vi "Save PDF files.vi"(6 "Duplicate Plot":bool, 7 "Open in Acrobat":bool, 9 "Desired Filename":string, 10 "Data Directories":string[](array[string]), 11 "PDF file in":path) -> (1 "Saved Files":path[](array[path]), 3 "Results Folders":path[](array[path]))   [LabVIEW 2021]
uses:
  Globals/Constants_global.vi
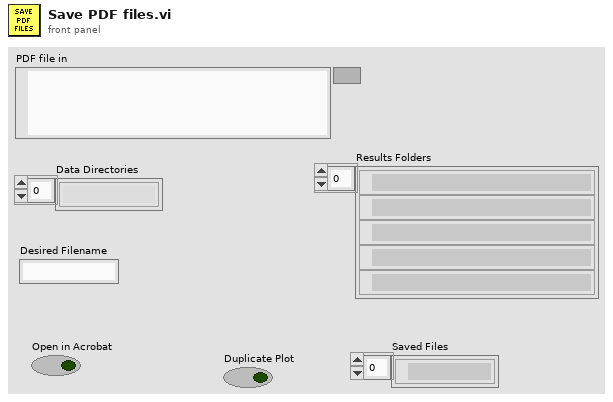
[diagram p1: front panel]
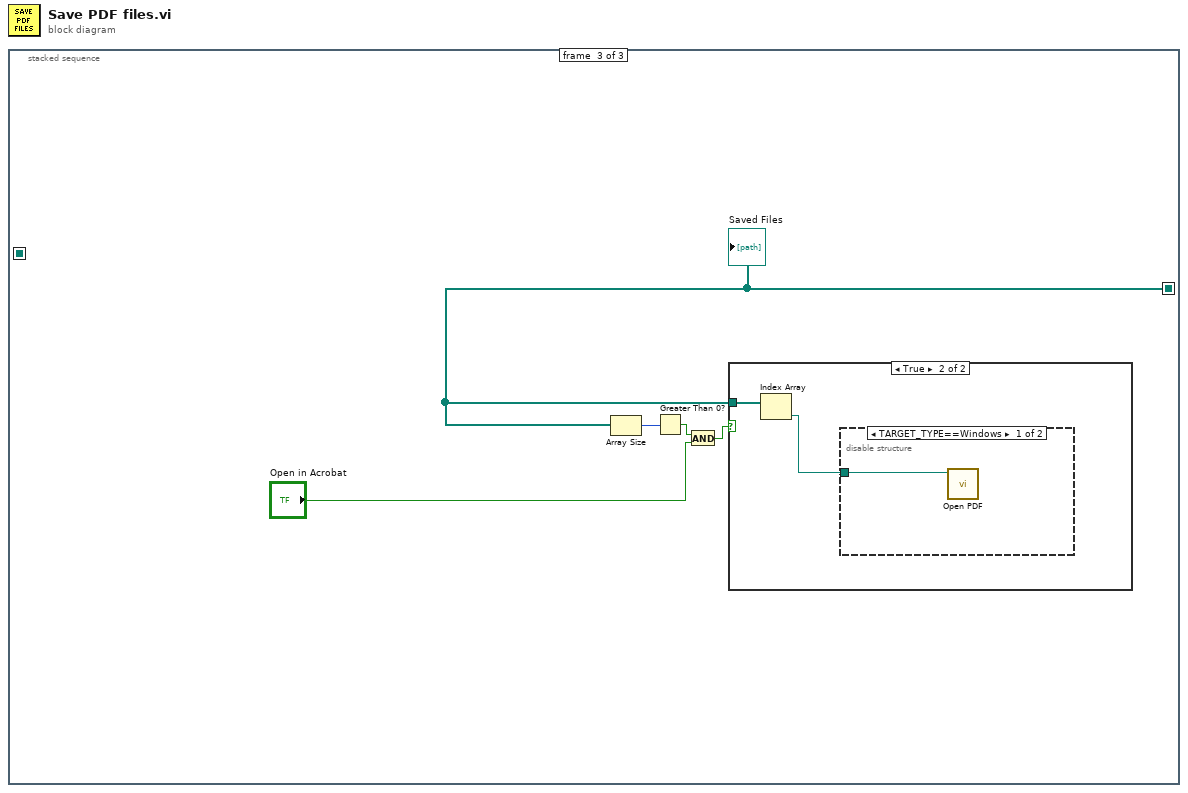
[diagram p0: block diagram]
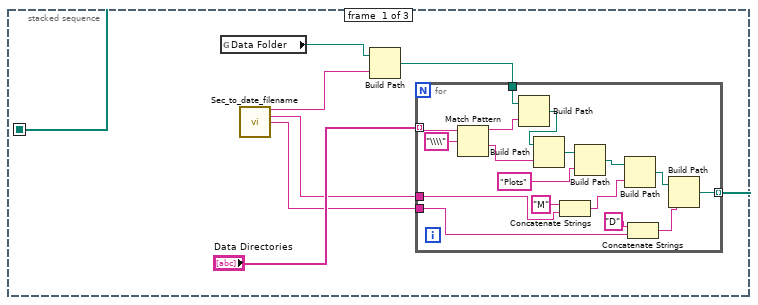
[diagram p2: hidden frame]
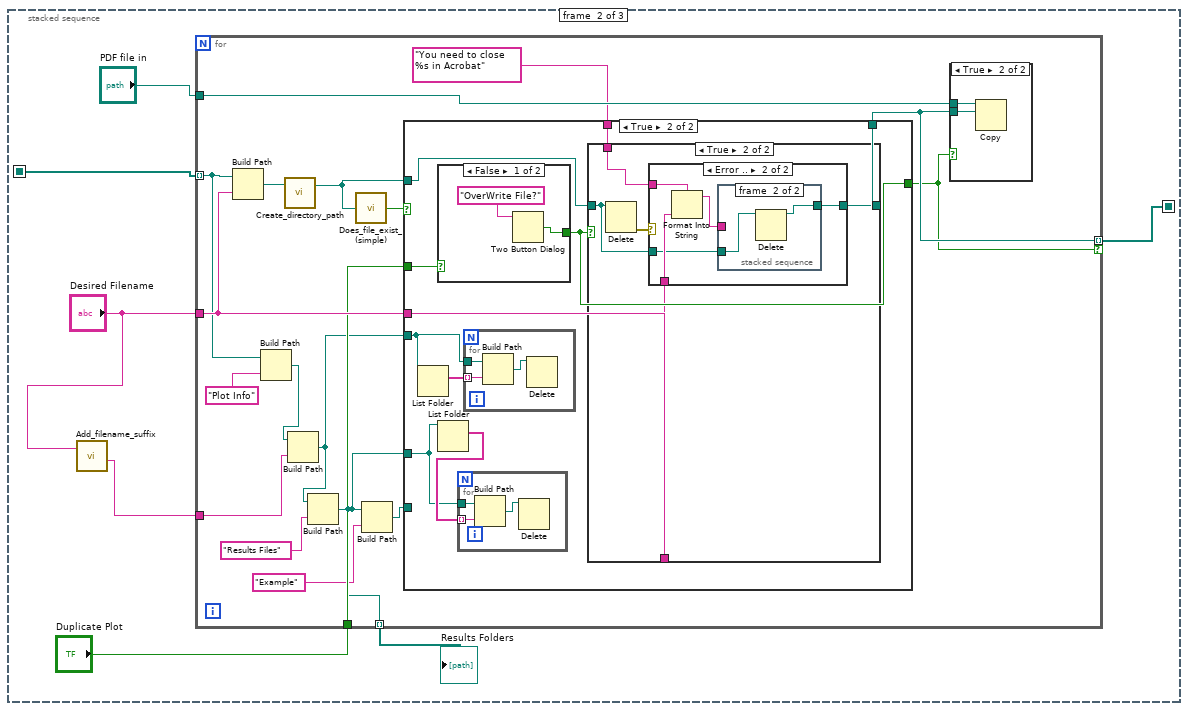
[diagram p3: hidden frame]
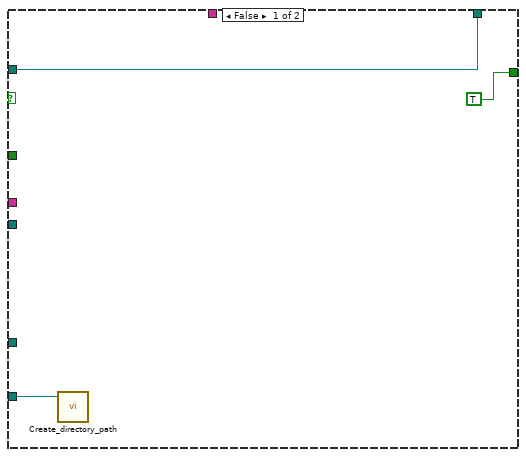
[diagram p5: hidden frame]
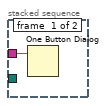
[diagram p8: hidden frame]
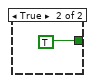
[diagram p9: hidden frame]
diagram:
  n1 = stacked-sequence {
    seq-local: [w3 _ _] -> [_ w29 _]
    seq-local: [_ w28 _] -> [_ _ w89]
    frame #0 {
      n2 = global read "Constants_global.vi" "Data Folder"() -> (w6:path)
      n3 = call "Sec_to_date_filename.vi"() -> ("YYYY"=w7:string, "mm-YYYY"=w1:string, "DD"=w2:string)  [unwired: 6 in, 7 out]
      n4 = Build Path(base path=w6, name or relative path=w7) -> (appended path=w5:path)
      n5 = for {
        tunnel: "Data Directories" -> [w24] mode=indexing
        tunnel: w5 -> [w22]
        tunnel: w1 -> [w13]
        tunnel: w2 -> [w10]
        tunnel: [w8] -> w3 mode=indexing
        n6 = Match Pattern(string=w24, regular expression="\\\\") -> (before substring=w20:string, after substring=w19:string)  [unwired: 1 in, 2 out]
        n7 = Build Path(base path=w22, name or relative path=w20) -> (appended path=w21:path)
        n8 = Build Path(base path=w21, name or relative path=w19) -> (appended path=w18:path)
        n9 = Concatenate Strings("M" ("string"), w13) -> (w15:string)
        n10 = Build Path(base path=w18, name or relative path="Plots") -> (appended path=w16:path)
        n11 = Build Path(base path=w16, name or relative path=w15) -> (appended path=w12:path)
        n12 = Concatenate Strings("D" ("string"), w10) -> (w9:string)
        n13 = Build Path(base path=w12, name or relative path=w9) -> (appended path=w8:path)
      }
    }
    frame #1 {
      n14 = call "Add_filename_suffix.vi"("Filename"="Desired Filename") -> ("Base name"=w25:string)  [unwired: 1 in, 3 out]
      n15 = for {
        tunnel: w29 -> [w40] mode=indexing
        tunnel: "Desired Filename" -> [w43]
        tunnel: "PDF file in" -> [w49]
        tunnel: [w45] -> w28 mode=indexing if=w44
        tunnel: "Duplicate Plot" -> [w41]
        tunnel: w25 -> [w37]
        tunnel: [w33] -> w27 mode=indexing
        n16 = Build Path(base path=w40, name or relative path=w43) -> (appended path=w48:path)
        n17 = Build Path(base path=w40, name or relative path="Plot Info") -> (appended path=w38:path)
        n18 = call "Create_directory_path.vi"("Path name"=w48) -> ("Path name Out"=w46:path)  [unwired: 2 in, 1 out]
        n19 = Build Path(base path=w38, name or relative path=w37) -> (appended path=w32:path)
        n20 = Build Path(base path=w32, name or relative path="Results Files") -> (appended path=w33:path)
        n21 = call "Does_file_exist_(simple).vi"("Pathname"=w46) -> ("exists?"=w47:bool)
        n22 = Build Path(base path=w33, name or relative path="Example") -> (appended path=w34:path)
        n23 = case shown="True" w47 {
          tunnel: [w54 w62] -> w45
          tunnel: w46 -> [w54 w63]
          tunnel: w41 -> [_ w64]
          tunnel: [TRUE w61] -> w44
          tunnel: w43 -> [_ w60]
          tunnel: "You need to close %s in Acrobat" ("message") -> [_ w59]
          tunnel: w34 -> [w52 _]
          tunnel: w33 -> [_ w57]
          tunnel: w32 -> [_ w56]
          frame False {
            n24 = call "Create_directory_path.vi"("Path name"=w52) -> ()  [unwired: 2 in, 2 out]
          }
          frame True {
            n25 = List Folder(path=w56) -> (filenames=w55:string[])  [unwired: 3 in, 3 out]
            n26 = case shown="False" w64 {
              tunnel: [w86 TRUE] -> w61
              frame False {
                n27 = Two Button Dialog(message="OverWrite File?") -> (T button?=w86:bool)  [unwired: 2 in]
              }
              frame True {
              }
            }
            n28 = List Folder(path=w57) -> (filenames=w58:string[])  [unwired: 3 in, 3 out]
            n29 = for {
              tunnel: w58 -> [w69] mode=indexing
              tunnel: w57 -> [w68]
              n30 = Build Path(base path=w68, name or relative path=w69) -> (appended path=w70:path)
              n31 = Delete(path (use dialog)=w70) -> ()  [unwired: 4 in, 3 out]
            }
            n32 = for {
              tunnel: w55 -> [w66] mode=indexing
              tunnel: w56 -> [w65]
              n33 = Build Path(base path=w65, name or relative path=w66) -> (appended path=w67:path)
              n34 = Delete(path (use dialog)=w67) -> ()  [unwired: 4 in, 3 out]
            }
            n35 = case shown="True" w61 {
              tunnel: w63 -> [w71 w74]
              tunnel: [w71 w73] -> w62
              tunnel: w60 -> [_ w75]
              tunnel: w59 -> [_ w72]
              frame False {
              }
              frame True {
                n36 = Delete(path (use dialog)=w74) -> (error out=w76:errorcluster)  [unwired: 4 in, 2 out]
                n37 = case shown="Error .." w76 {
                  tunnel: w75 -> [_ w82]
                  tunnel: w74 -> [w77 w80]
                  tunnel: [w77 w79] -> w73
                  tunnel: w72 -> [_ w78]
                  frame No Error {
                  }
                  frame Error {
                    n38 = Format Into String(format string=w78, w82) -> (resulting string=w81:string)  [unwired: 2 in, 1 out]
                    n39 = stacked-sequence {
                      tunnel: w81 -> [w83 _]
                      tunnel: w80 -> [_ w85]
                      tunnel: [_ w84] -> w79
                      frame #0 {
                        n40 = One Button Dialog(message=w83) -> ()  [unwired: 1 in, 1 out]
                      }
                      frame #1 {
                        n41 = Delete(path (use dialog)=w85) -> (deleted path=w84:path)  [unwired: 4 in, 2 out]
                      }
                    }
                  }
                }
              }
            }
          }
        }
        n42 = case shown="True" w44 {
          tunnel: w49 -> [_ w51]
          tunnel: w45 -> [_ w50]
          frame False {
          }
          frame True {
            n43 = Copy(10:w50, 11:w51) -> ()  [unwired: 3 in, 3 out]
          }
        }
      }
      "Results Folders" <- w27
    }
    frame #2 {
      n44 = Array Size(array=w89) -> (size(s)=w92:i32)
      n45 = Greater Than 0?(x=w92) -> (x > 0?=w91:bool)
      n46 = And(x=w91, y="Open in Acrobat") -> (x .and. y?=w90:bool)
      n47 = case shown="True" w90 {
        tunnel: w89 -> [_ w95]
        frame False {
        }
        frame True {
          n48 = Index Array(array=w95) -> (element=w94:path)  [unwired: 1 in]
          n49 = disable-structure shown="TARGET_TYPE==Windows" {
            disable-tunnel: w94 -> [w96 _]
            frame condition #0 (active) {
              n50 = call "Open PDF.vi"("Path"=w96) -> ()  [unwired: 5 in, 2 out]
            }
            frame condition #1 {
            }
          }
        }
      }
      "Saved Files" <- w89
    }
  }
